vi "Display Pop Up.vi"(9 "Display time out(-1ms)":i32=-1, 10 "Content":string, 11 "Header":string) -> ()   [LabVIEW 2020, in "Msg.lvlib"]
uses:
  Msg.lvlib
panel:
  out "String":string
  in  "OK":bool
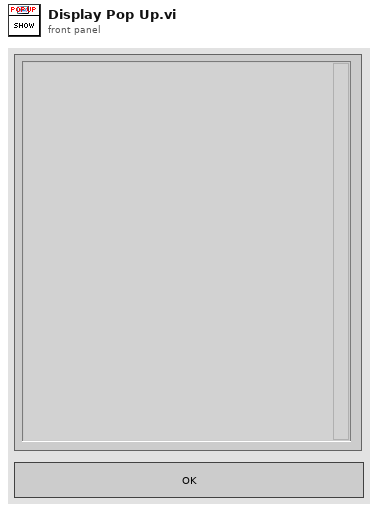
[diagram p1: front panel]
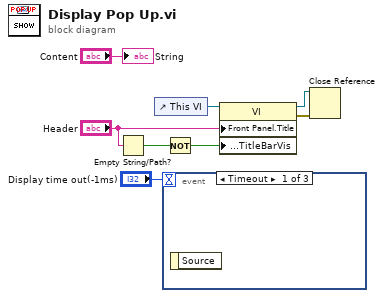
[diagram p0: block diagram]
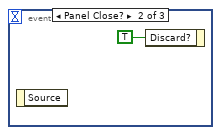
[diagram p2: hidden frame]
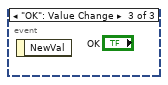
[diagram p3: hidden frame]
diagram:
  n1 = Empty String/Path?(string/path="Header") -> (empty?=w5:bool)
  n2 = control-ref of="This VI"() -> (w7:refnum<vi>)
  n3 = event shown="[0] Timeout" {
    selector: _ -> [_ _ _]
    dyn-events: _ -> [_ _ _]
    timeout: "Display time out(-1ms)" -> [_ _ _]
    event Timeout {
      n4 = event-data() -> ()  [unwired: 1 in, 1 out]
    }
    event Panel Close? {
      n5 = event-data() -> ()  [unwired: 1 in, 1 out]
      n6 = event-data("Discard?"=TRUE) -> ()  [unwired: 1 in, 1 out]
    }
    event "OK": Value Change {
      n7 = event-data() -> ()  [unwired: 1 in, 1 out]
    }
  }
  n8 = Not(x=w5) -> (.not. x?=w4:bool)
  n9 = property class="VI"(reference=w7, "Front Panel.Title"="Header", "Front Panel.TitleBarVis"=w4) -> (reference out=w2:refnum<vi>, error out=w3:errorcluster)  [unwired: 1 in]
  n10 = Close Reference(reference=w2, error in (no error)=w3) -> ()  [unwired: 1 out]
  "String" <- "Content"
